vi "CheckAlarms.vi"(10 "Values":dbl[](array[numeric]), 11 "Alarm Setups":T2[](array[typedef])) -> (2 "Alarm Tripped?":bool, 3 "Alarm Data":T1[](array[typedef]))   [LabVIEW 2012]
uses:
  AlarmSetup.ctl
  AlarmDatum.ctl
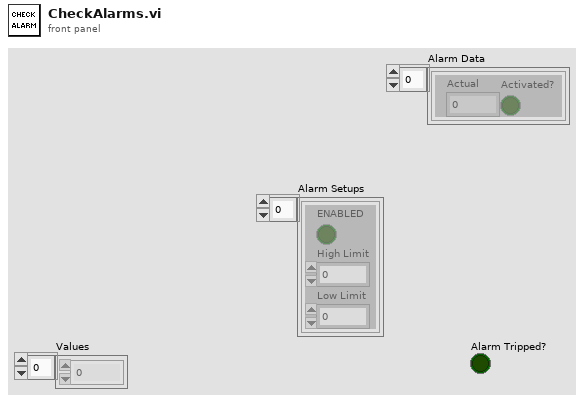
[diagram p1: front panel]
types:
  T1 = typedef "AlarmDatum.ctl" = cluster{"Actual":dbl, "Activated?":bool}
  T2 = typedef "AlarmSetup.ctl" = cluster{"ENABLED":bool, "High Limit":dbl, "Low Limit":dbl}
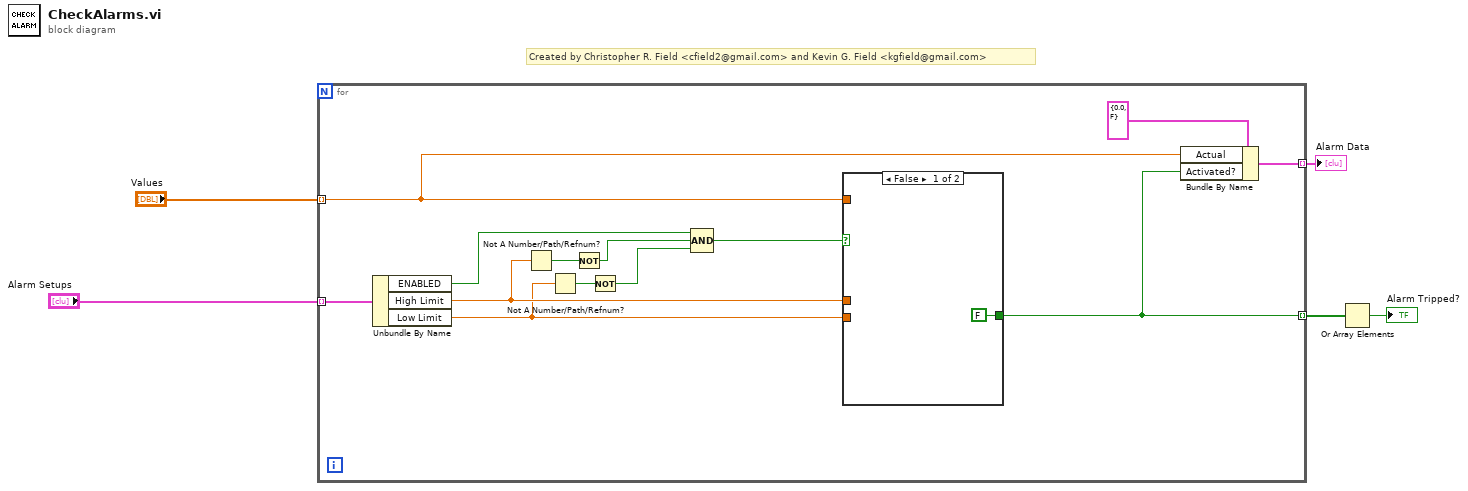
[diagram p0: block diagram]
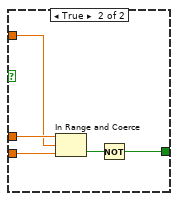
[diagram p2: hidden frame]
diagram:
  # "Created by Christopher R. Field <cfield2@gmail.com> and Kevin G. Field <kgfield@gmail.com>"
  n1 = for {
    tunnel: "Values" -> [w17] mode=indexing
    tunnel: "Alarm Setups" -> [w18] mode=indexing
    tunnel: [w16] -> w1 mode=indexing
    tunnel: [w15] -> w4 mode=indexing
    n2 = Unbundle By Name(w18) -> ("ENABLED"=w14:bool, "High Limit"=w13:dbl, "Low Limit"=w10:dbl)
    n3 = Not A Number/Path/Refnum?(number/path/refnum=w13) -> (NaN/Path/Refnum?=w12:bool)
    n4 = Not A Number/Path/Refnum?(number/path/refnum=w10) -> (NaN/Path/Refnum?=w9:bool)
    n5 = Not(x=w12) -> (.not. x?=w11:bool)
    n6 = Not(x=w9) -> (.not. x?=w8:bool)
    n7 = Compound Arithmetic op=AND(w14, w11, w8) -> (w7:bool)
    n8 = case shown="False" w7 {
      tunnel: w17 -> [_ w22]
      tunnel: w13 -> [_ w24]
      tunnel: w10 -> [_ w23]
      tunnel: [FALSE w20] -> w15
      frame False {
      }
      frame True {
        n9 = In Range and Coerce(upper limit=w24, x=w22, lower limit=w23) -> (In Range?=w21:bool)  [unwired: 1 out]
        n10 = Not(x=w21) -> (.not. x?=w20:bool)
      }
    }
    n11 = Bundle By Name(cluster=T1 {"Actual"=0.0, "Activated?"=FALSE} ("Alarm Datum"), "Actual"=w17, "Activated?"=w15) -> (w16:T1)
  }
  "Alarm Data" <- w1
  n12 = Or Array Elements(Boolean array=w4) -> (logical OR=→"Alarm Tripped?":bool)
